vi "open connection.vi"(8 "error in (no error)":errorcluster caption="Fehler (Eingang, kein Fehler)", 11 "Tektronix RSA5106A Eingang":refnum<class "Tektronix RSA5106A.lvclass"> caption="DNL_LabVIEW Object in") -> (0 "error out":errorcluster caption="Fehler (Ausgang)", 3 "Tektronix RSA5106A Ausgang":refnum<class "Tektronix RSA5106A.lvclass"> caption="DNL_LabVIEW Object out")   [LabVIEW 2013, in "Tektronix RSA5106A.lvclass"]
uses:
  Tektronix RSA5106A.lvclass
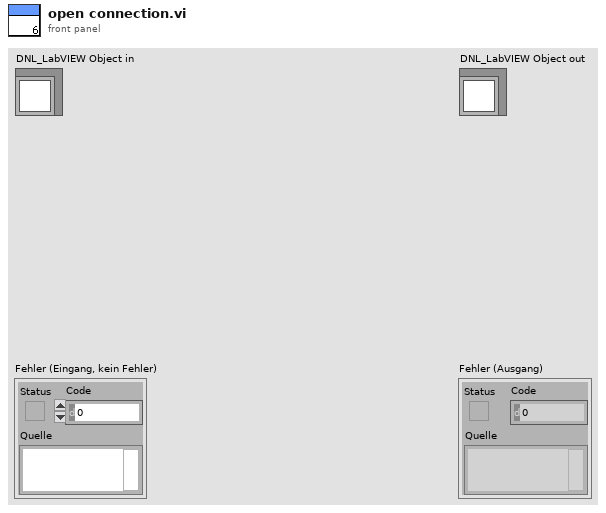
[diagram p1: front panel]
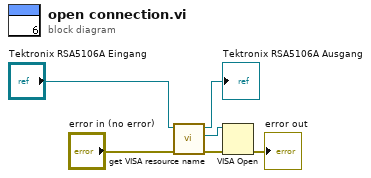
[diagram p0: block diagram]
diagram:
  n1 = call-dynamic "get VISA resource name.vi"("error in (no error)"="error in (no error)", "DeviceInterface (Eingang)"="Tektronix RSA5106A Eingang") -> ("error out"=w2:errorcluster, "VISA resource name"=w3:refnum<visa-resource-name>, "DeviceInterface (Ausgang)"=→"Tektronix RSA5106A Ausgang":refnum<class "Tektronix RSA5106A.lvclass">)  [unwired: 7 in]
  n2 = VISA Open(error in (no error)=w2, VISA resource name=w3) -> (error out=→"error out":errorcluster)  [unwired: 3 in, 1 out]
